vi "LAUNCH Rigol DG822 Square.vi"   [LabVIEW 2021]
uses:
  General/Files/lvlibp/Actors.lvlibp/Actors/Actors/Actors.lvclass
panel:
  # "Launch Rigol DG822 Square"
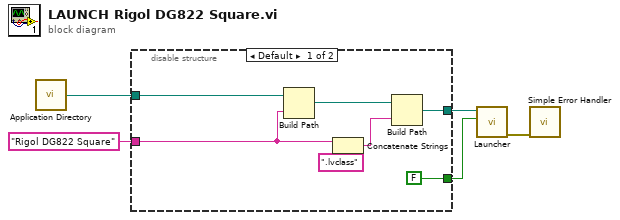
[diagram p0: block diagram]
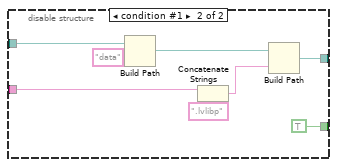
[diagram p2: hidden frame]
diagram:
  n1 = call <vilib>:"Application Directory.vi"() -> ("Application Directory"=w1:path)
  n2 = disable-structure shown="Default" {
    disable-tunnel: [w12 w18] -> w3
    disable-tunnel: w1 -> [w6 w17]
    disable-tunnel: "Rigol DG822 Square" ("concatenated string") -> [w7 w16]
    disable-tunnel: [FALSE TRUE] -> w2
    frame condition #0 (active) {
      n3 = Build Path(base path=w6, name or relative path=w7) -> (appended path=w8:path)
      n4 = Concatenate Strings(w7, ".lvclass" ("name or relative path")) -> (w10:string)
      n5 = Build Path(base path=w8, name or relative path=w10) -> (appended path=w12:path)
    }
    frame condition #1 {
      n6 = Build Path(base path=w17, name or relative path="data") -> (appended path=w20:path)
      n7 = Concatenate Strings(w16, ".lvlibp" ("name or relative path")) -> (w14:string)
      n8 = Build Path(base path=w20, name or relative path=w14) -> (appended path=w18:path)
    }
  }
  n9 = call "Launcher.vi"("is exe?"=w2, "packed library path"=w3) -> ("Error"=w4:errorcluster)  [unwired: 8 in, 1 out]
  n10 = call <vilib>:"Simple Error Handler.vi"("error in (no error)"=w4) -> ()  [unwired: 4 in, 5 out]
